vi "Motor2DLaserScan.vi"() -> ()   [LabVIEW 2017]
doc: "2D motor scan example Vi."
uses:
  C:/Users/apresyan/Laser2DScan/Thorlabs.MotionControl.Controls.dll
  Thorlabs.MotionControl.Controls.dll
  C:/Users/apresyan/Laser2DScan/Thorlabs.MotionControl.Benchtop.StepperMotorCLI.dll
  Thorlabs.MotionControl.Benchtop.StepperMotorCLI.dll
  C:/Users/apresyan/Laser2DScan/Thorlabs.MotionControl.IntegratedStepperMotorsCLI.dll
  Thorlabs.MotionControl.IntegratedStepperMotorsCLI.dll
panel:
  in  "Step Size Y (mm)":sgl=0.25 format="%.2f"
  in  "Num Of Steps X":i32=4
  in  "X Start Position":sgl
  in  "Y Start Position":sgl
  in  "Num Of Steps Y":i32=4
  in  "Step Size X (mm)":sgl=0.25 format="%.2f"
  in  "Labjack Serial Number":string="49876934"
  in  "LabJackControl":refnum<k24>(container)
  in  "BenchtopStepperControl":refnum<k24>(container)
  in  "Benchtop SerialNumber":string="70876766"
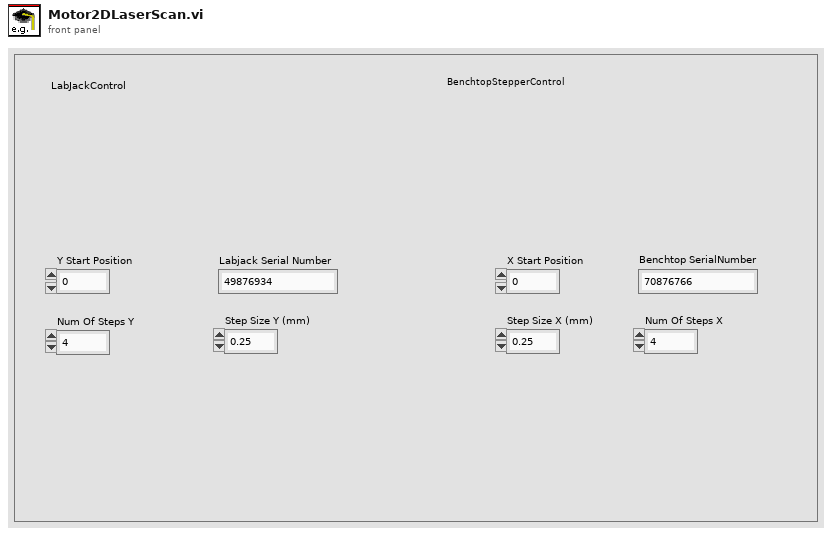
[diagram p1: front panel]
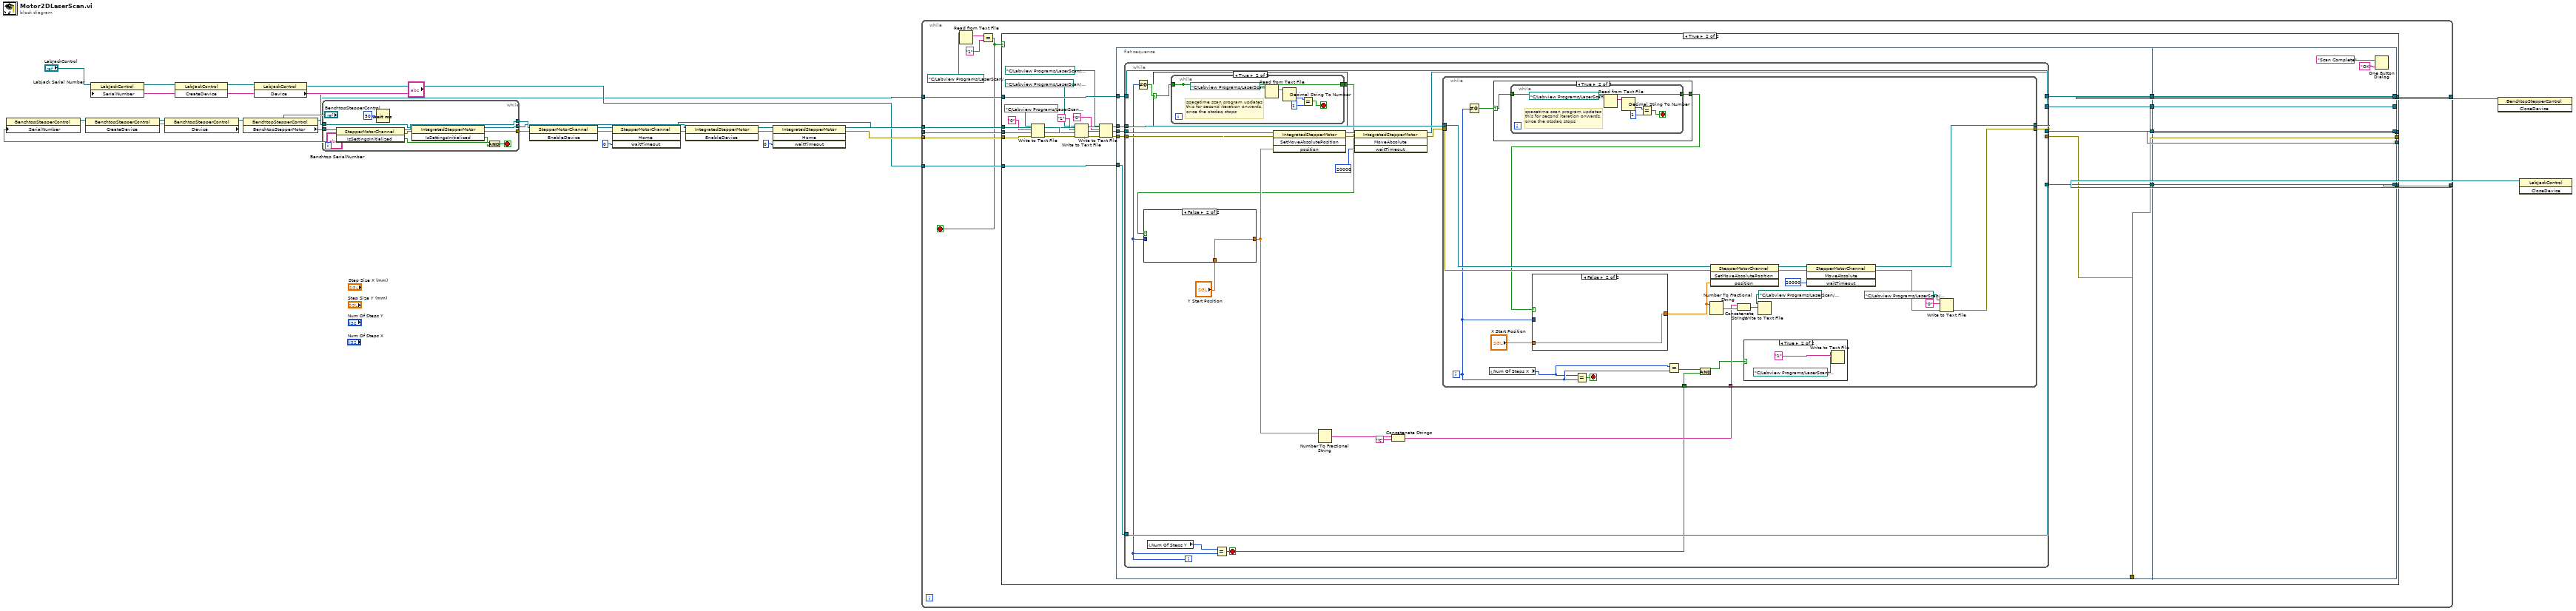
[diagram p0: block diagram]
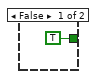
[diagram p3: hidden frame]
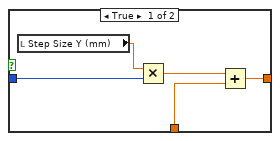
[diagram p4: hidden frame]
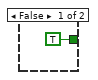
[diagram p6: hidden frame]
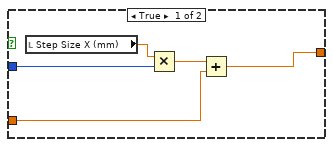
[diagram p7: hidden frame]
diagram:
  n1 = property class="BenchtopStepperControl"(reference="BenchtopStepperControl", "SerialNumber"="Benchtop SerialNumber") -> (reference out=w26:refnum<k24>)  [unwired: 1 in, 1 out]
  n2 = invoke class="BenchtopStepperControl" method="CreateDevice"(reference=w26) -> (reference out=w24:refnum<k24>, error out=w27:errorcluster)  [unwired: 2 in, 1 out]
  n3 = property class="LabJackControl"(reference="LabJackControl", "SerialNumber"="Labjack Serial Number") -> (reference out=w14:refnum<k24>)  [unwired: 1 in, 1 out]
  n4 = property class="BenchtopStepperControl" props=["Device"](reference=w24, error in=w27) -> (reference out=w25:refnum<k24>)  [unwired: 2 out]
  n5 = invoke class="LabJackControl" method="CreateDevice"(reference=w14) -> (reference out=w13:refnum<k24>)  [unwired: 2 in, 2 out]
  n6 = property class="BenchtopStepperControl"(reference=w25) -> (reference out=w1:refnum<k24>, "BenchtopStepperMotor"=w11:refnum<k24>)  [unwired: 1 in, 1 out]
  n7 = property class="LabJackControl"(reference=w13) -> (reference out=w2:refnum<k24>, "Device"=w12:refnum<k24>)  [unwired: 1 in, 1 out]
  n8 = while {
    tunnel: [w36] -> w10
    tunnel: [w35] -> w9
    tunnel: [w33] -> w8
    tunnel: w12 -> [w31]
    tunnel: w11 -> [w30]
    stop <- w37 stop-if-true
    n9 = invoke class="StepperMotorChannel" method="IsSettingsInitialized"(reference=w30) -> (reference out=w36:refnum<k24>, error out=w32:errorcluster, "IsSettingsInitialized"=w39:bool)  [unwired: 2 in]
    n10 = Wait (ms)(milliseconds to wait=u32 50) -> ()  [unwired: 1 out]
    n11 = invoke class="IntegratedStepperMotor" method="IsSettingsInitialized"(reference=w31, error in=w32) -> (reference out=w35:refnum<k24>, error out=w33:errorcluster, "IsSettingsInitialized"=w38:bool)  [unwired: 1 in]
    n12 = And(x=w39, y=w38) -> (x .and. y?=w37:bool)
  }
  n13 = invoke class="StepperMotorChannel" method="EnableDevice"(reference=w10, error in=w8) -> (reference out=w21:refnum<k24>, error out=w19:errorcluster)  [unwired: 1 in, 1 out]
  n14 = invoke class="StepperMotorChannel" method="Home"(reference=w21, error in=w19, "waitTimeout"=0) -> (reference out=w4:refnum<k24>, error out=w17:errorcluster)  [unwired: 1 in, 2 out]
  n15 = invoke class="IntegratedStepperMotor" method="EnableDevice"(reference=w9, error in=w17) -> (reference out=w20:refnum<k24>, error out=w18:errorcluster)  [unwired: 1 in, 1 out]
  n16 = invoke class="IntegratedStepperMotor" method="Home"(reference=w20, error in=w18, "waitTimeout"=0) -> (reference out=w3:refnum<k24>, error out=w5:errorcluster)  [unwired: 1 in, 2 out]
  n17 = while {
    tunnel: w3 -> [w50]
    tunnel: w5 -> [w48]
    tunnel: w4 -> [w49]
    tunnel: w2 -> [w47]
    tunnel: w1 -> [w46]
    tunnel: [w45] -> w7
    tunnel: [w44] -> w6
    stop <- w40 stop-if-true
    n18 = Read from Text File(file (use dialog)=path "C:/Labview Programs/LaserScan/MotorControlTextFiles/ScanInitiate.txt") -> (text=w41:string)  [unwired: 3 in, 3 out]
    n19 = Equal?(x=w41, y="1") -> (x = y?=w40:bool)
    n20 = case shown="True" w40 {
      tunnel: [w55 w78] -> _
      tunnel: [w54 w77] -> _
      tunnel: w49 -> [w54 w76]
      tunnel: w50 -> [w55 w75]
      tunnel: w48 -> [w53 w63]
      tunnel: [w53 w72] -> _
      tunnel: w47 -> [w52 w71]
      tunnel: w46 -> [w51 w70]
      tunnel: [w52 w69] -> w45
      tunnel: [w51 w67] -> w44
      frame False {
      }
      frame True {
        n21 = Write to Text File(file (use dialog)=path "C:/Labview Programs/LaserScan/MotorControlTextFiles/ScanInitiate.txt" ("file path (use dialog)"), text="0", error in=w63) -> (error out=w57:errorcluster)  [unwired: 1 in, 2 out]
        n22 = Write to Text File(file (use dialog)=path "C:/Labview Programs/LaserScan/MotorControlTextFiles/MotorReadyToMove.txt" ("file path (use dialog)"), text="1", error in=w57) -> (error out=w58:errorcluster)  [unwired: 1 in, 2 out]
        n23 = Write to Text File(file (use dialog)=path "C:/Labview Programs/LaserScan/MotorControlTextFiles/LastIterationBool.txt" ("file path (use dialog)"), text="0", error in=w58) -> (error out=w56:errorcluster)  [unwired: 1 in, 2 out]
        n24 = flat-sequence {
          tunnel: w76 -> [w86]
          tunnel: w75 -> [w85]
          tunnel: [w88] -> w74
          tunnel: [w87] -> w73
          tunnel: w56 -> [w84]
          tunnel: [w79] -> w72
          tunnel: w71 -> [w83]
          tunnel: w70 -> [w82]
          tunnel: [w81] -> w68
          tunnel: [w80] -> w66
          tunnel: [w171] -> w77
          tunnel: [w172] -> w78
          tunnel: w74 -> [w172]
          tunnel: w73 -> [w171]
          tunnel: [w168] -> w69
          tunnel: w68 -> [w168]
          tunnel: [w167] -> w67
          tunnel: w66 -> [w167]
          frame #0 {
            n25 = while {
              tunnel: w85 -> [w108]
              tunnel: w86 -> [w107]
              tunnel: [w105] -> w88
              tunnel: [w104] -> w87
              tunnel: w84 -> [w102]
              tunnel: [w100] -> w79
              tunnel: [w99] -> w81
              tunnel: w83 -> [w99]
              tunnel: [w98] -> w80
              tunnel: w82 -> [w98]
              i -> [w93]
              stop <- w90 stop-if-true
              n26 = Not Equal To 0?(x=w93) -> (x != 0?=w91:bool)
              n27 = local read "Num Of Steps Y"() -> (w110:i32)
              n28 = case shown="True" w91 {
                selector: w91 -> [_ w112]
                tunnel: [TRUE w113] -> w92
                frame False {
                }
                frame True {
                  n29 = while {
                    tunnel: w112 -> [w114]
                    tunnel: [w114] -> _
                    tunnel: [w114] -> w113
                    stop <- w115 stop-if-true
                    # "spacetime scan program updates this for second iteration onwards, once the otsdaq stops"
                    n30 = Read from Text File(file (use dialog)=path "C:/Labview Programs/LaserScan/MotorControlTextFiles/MotorReadyToMove.txt") -> (text=w118:string)  [unwired: 3 in, 3 out]
                    n31 = Decimal String To Number(string=w118) -> (number=w117:i32)  [unwired: 2 in, 1 out]
                    n32 = Equal?(x=w117, y=1) -> (x = y?=w115:bool)
                  }
                }
              }
              n33 = case shown="False" w92 {
                tunnel: [w122 w125] -> w97
                tunnel: w93 -> [w121 _]
                tunnel: "Y Start Position" -> [w120 w125]
                frame True {
                  n34 = local read "Step Size Y (mm)"() -> (w124:sgl)
                  n35 = Multiply(x=w124, y=w121) -> (x*y=w123:sgl)
                  n36 = Add(x=w123, y=w120) -> (x+y=w122:sgl)
                }
                frame False {
                }
              }
              n37 = Equal?(x=w110, y=w93) -> (x = y?=w90:bool)
              n38 = invoke class="IntegratedStepperMotor" method="SetMoveAbsolutePosition"(reference=w108, error in=w102, "position"=w97) -> (reference out=w109:refnum<k24>, error out=w103:errorcluster)  [unwired: 1 in, 2 out]
              n39 = Number To Fractional String(number=w97) -> (F-format string=w96:string)  [unwired: 3 in]
              n40 = invoke class="IntegratedStepperMotor" method="MoveAbsolute"(reference=w109, error in=w103, "waitTimeout"=20000) -> (reference out=w105:refnum<k24>, error out=w101:errorcluster)  [unwired: 1 in, 2 out]
              n41 = Concatenate Strings(w96, "\t") -> (w94:string)
              n42 = while {
                tunnel: w107 -> [w148]
                tunnel: [w146] -> w104
                tunnel: w101 -> [w145]
                tunnel: [w128] -> w100
                tunnel: w94 -> [w136]
                tunnel: w90 -> [w130]
                i -> [w132]
                stop <- w134 stop-if-true
                n43 = Not Equal To 0?(x=w132) -> (x != 0?=w133:bool)
                n44 = local read "Num Of Steps X"() -> (w126:i32)
                n45 = case shown="True" w133 {
                  selector: w133 -> [_ w153]
                  tunnel: [TRUE w154] -> w135
                  frame False {
                  }
                  frame True {
                    n46 = while {
                      tunnel: w153 -> [w155]
                      tunnel: [w155] -> w154
                      stop <- w156 stop-if-true
                      # "spacetime scan program updates this for second iteration onwards, once the otsdaq stops"
                      n47 = Read from Text File(file (use dialog)=path "C:/Labview Programs/LaserScan/MotorControlTextFiles/MotorReadyToMove.txt") -> (text=w159:string)  [unwired: 3 in, 3 out]
                      n48 = Decimal String To Number(string=w159) -> (number=w158:i32)  [unwired: 2 in, 1 out]
                      n49 = Equal?(x=w158, y=1) -> (x = y?=w156:bool)
                    }
                  }
                }
                n50 = case shown="False" w135 {
                  tunnel: [w163 w166] -> w140
                  tunnel: w132 -> [w162 _]
                  tunnel: "X Start Position" -> [w161 w166]
                  frame True {
                    n51 = local read "Step Size X (mm)"() -> (w165:sgl)
                    n52 = Multiply(x=w165, y=w162) -> (x*y=w164:sgl)
                    n53 = Add(x=w164, y=w161) -> (x+y=w163:sgl)
                  }
                  frame False {
                  }
                }
                n54 = Equal?(x=w126, y=w132) -> (x = y?=w134:bool)
                n55 = Equal?(x=w126, y=w132) -> (x = y?=w131:bool)
                n56 = And(x=w131, y=w130) -> (x .and. y?=w129:bool)
                n57 = Number To Fractional String(number=w140) -> (F-format string=w137:string)  [unwired: 3 in]
                n58 = invoke class="StepperMotorChannel" method="SetMoveAbsolutePosition"(reference=w148, error in=w145, "position"=w140) -> (reference out=w149:refnum<k24>, error out=w144:errorcluster)  [unwired: 1 in, 2 out]
                n59 = Concatenate Strings(w136, w137) -> (w139:string)
                n60 = case shown="True" w129 {
                  frame False {
                  }
                  frame True {
                    n61 = Write to Text File(file (use dialog)=path "C:/Labview Programs/LaserScan/MotorControlTextFiles/LastIterationBool.txt" ("file path (use dialog)"), text="1") -> ()  [unwired: 2 in, 3 out]
                  }
                }
                n62 = Write to Text File(file (use dialog)=path "C:/Labview Programs/LaserScan/MotorControlTextFiles/Motor2DPosition.txt" ("file path (use dialog)"), text=w139) -> ()  [unwired: 2 in, 3 out]
                n63 = invoke class="StepperMotorChannel" method="MoveAbsolute"(reference=w149, error in=w144, "waitTimeout"=20000) -> (reference out=w146:refnum<k24>, error out=w143:errorcluster)  [unwired: 1 in, 2 out]
                n64 = Write to Text File(file (use dialog)=path "C:/Labview Programs/LaserScan/MotorControlTextFiles/MotorReadyToMove.txt" ("file path (use dialog)"), text="0", error in=w143) -> (error out=w128:errorcluster)  [unwired: 1 in, 2 out]
              }
            }
          }
          frame #1 {
            n65 = One Button Dialog(message="Scan Complete", button name ("OK")="OK") -> ()  [unwired: 1 out]
          }
        }
      }
    }
  }
  n66 = invoke class="BenchtopStepperControl" method="CloseDevice"(reference=w6) -> ()  [unwired: 2 in, 3 out]
  n67 = invoke class="LabJackControl" method="CloseDevice"(reference=w7) -> ()  [unwired: 2 in, 3 out]
